vi "AIMeasureVoltage.vi"(9 "Min Voltage":dbl=-10.0, 10 "Max Voltage":dbl=10.0, 11 "Physical Channel":tag="DAQ/ai0") -> (0 "error out":errorcluster, 3 "Voltage":dbl format="%0.2f")   [LabVIEW 2012]
uses:
  <vilib>/DAQmx/read.llb/DAQmx Read (Analog DBL 1Chan 1Samp).vi
  <vilib>/DAQmx/create/channels.llb/DAQmx Create Channel (AI-Voltage-Basic).vi
  <vilib>/DAQmx/miscellaneous.llb/DAQmx Fill In Error Info.vi
panel:
  # "Channel Settings"
  # "Results"
  # "Acquired Data"
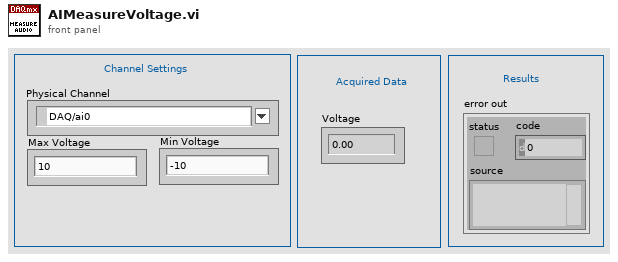
[diagram p1: front panel]
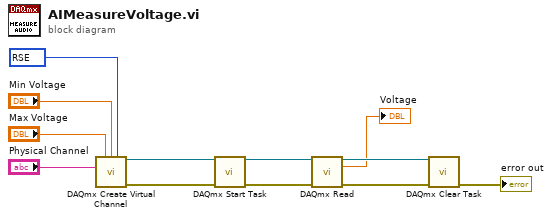
[diagram p0: block diagram]
diagram:
  w7 = 10083 items=["default"=-1, "RSE"=10083, "NRSE"=10078, "Differential"=10106, "Pseudodifferential"=12529] ("input terminal configuration")
  n1 = call-poly <vilib>:"DAQmx Create Virtual Channel.vi"("maximum value"="Max Voltage", "minimum value"="Min Voltage", "input terminal configuration"=w7, "physical channels"="Physical Channel") -> ("task out"=w3:refnum<k21>, "error out"=w2:errorcluster)  [unwired: 10 in]
  n2 = call <vilib>:"DAQmx Start Task.vi"("task/channels in"=w3, "error in"=w2) -> ("task out"=w12:refnum<k21>, "error out"=w11:errorcluster)  [unwired: 12 in]
  n3 = call-poly <vilib>:"DAQmx Read.vi"("task/channels in"=w12, "error in"=w11) -> ("task out"=w10:refnum<k21>, "data"=→"Voltage":dbl, "error out"=w9:errorcluster)  [unwired: 11 in]
  n4 = call <vilib>:"DAQmx Clear Task.vi"("task in"=w10, "error in"=w9) -> ("error out"=→"error out":errorcluster)  [unwired: 13 in]
